vi "Mirror_Scan_Pixels_Main_V2.vi"() -> ()   [LabVIEW 2014]
uses:
  Pixel Scan Parameters.ctl
  MirrorModes.ctl
  Standard Action.ctl
  <vilib>/Analysis/baseanly.llb/Mean (DBL).vi
  <vilib>/Utility/file.llb/Write To Spreadsheet File (DBL).vi
  <vilib>/Utility/file.llb/Read From Spreadsheet File (DBL).vi
  <vilib>/Analysis/NI_AALBase.lvlib
panel:
  in  "Apply Zero":bool
  in  "Load V Map":bool
  in  "Load Modes":bool
  in  "Save Modes":bool
  in  "Save V Map":bool
  in  "Apply Flat":bool
  in  "Center Bias":bool
  in  "Exit":bool
  in  "Mirror Tab":T1(tab)
  in  "Mirror Modes":T2
  in  "Pixel Scan Parameters":T3={"Scan Start Pixel"=1, "Scan End Pixel"=1, "Pixel Start Value (-1 to 1)"=-0.5, "Pixel End Value (-1 to 1)"=0.5, "Number of Steps"=0.1}
  in  "Start Pixel Scan":bool
  out "Pixel Map (-1 to 1)":dbl[][](graph)
  # "Mode"
  # "Amount (nm)"
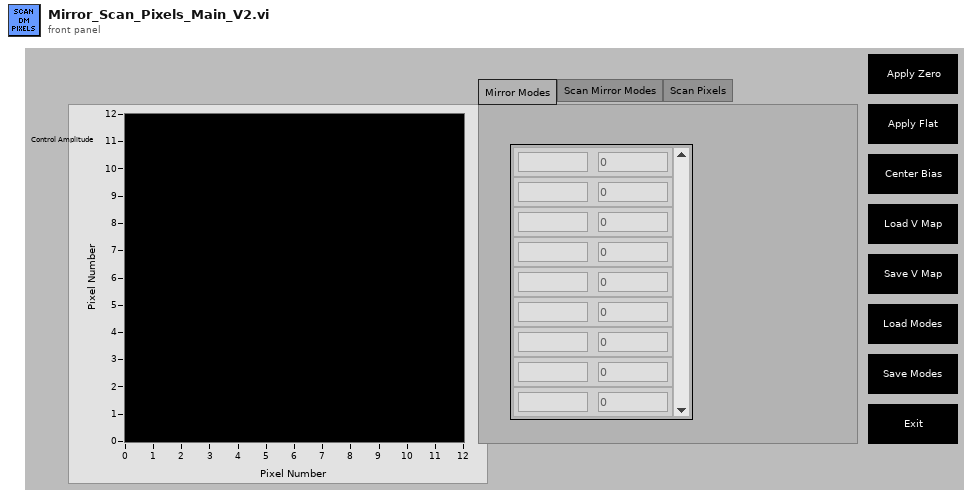
[diagram p1: front panel]
types:
  T1 = enum32{"Mirror Modes", "Scan Mirror Modes", "Scan Pixels"}
  T2 = typedef "MirrorModes.ctl" = cluster{"Mode":string, "Amplitude":dbl}[]
  T3 = typedef "Pixel Scan Parameters.ctl" = cluster{"Scan Start Pixel":i32, "Scan End Pixel":i32, "Pixel Start Value (-1 to 1)":dbl, "Pixel End Value (-1 to 1)":dbl, "Number of Steps":dbl}
  T4 = enum16{"Start Scan", "Reset Counter", "Write DM", "Get Image", "Update Count", "Exit"}
  T5 = typedef "Standard Action.ctl" = enum16{"Read", "Write"}
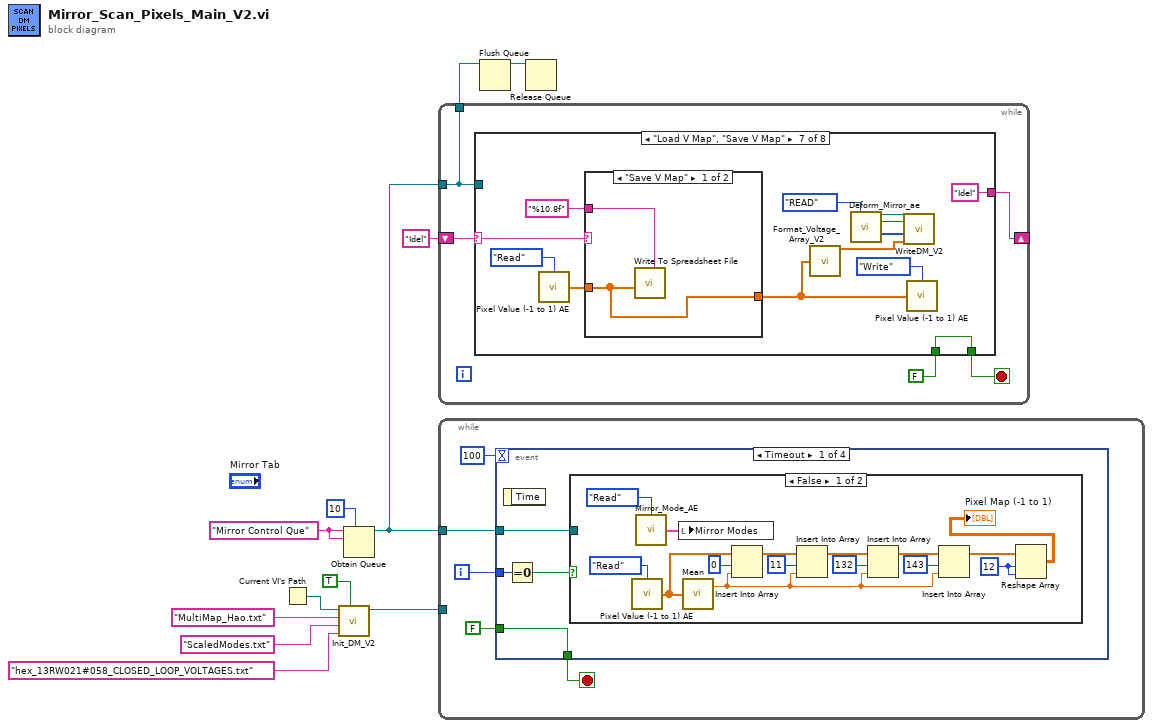
[diagram p0: block diagram]
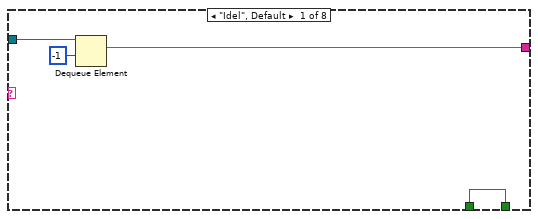
[diagram p2: hidden frame]
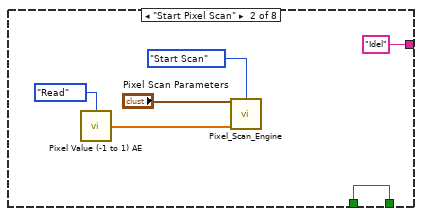
[diagram p3: hidden frame]
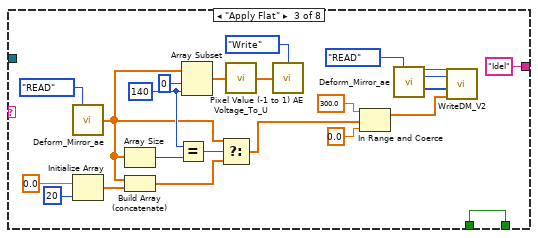
[diagram p4: hidden frame]
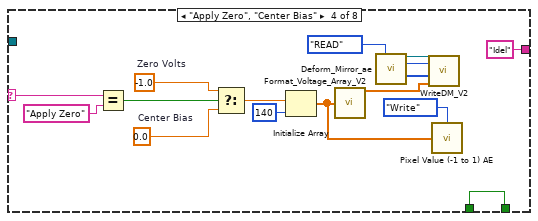
[diagram p5: hidden frame]
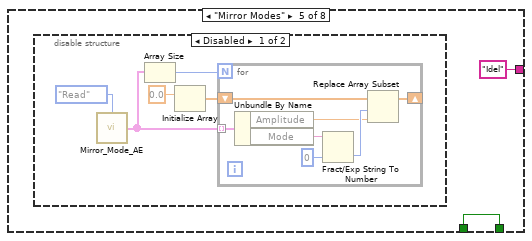
[diagram p6: hidden frame]
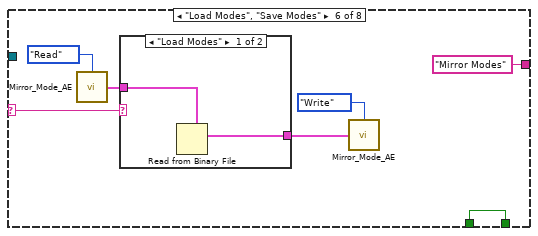
[diagram p8: hidden frame]
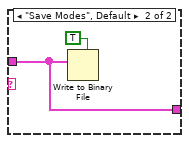
[diagram p9: hidden frame]
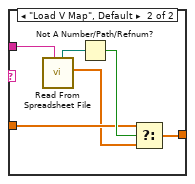
[diagram p10: hidden frame]
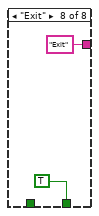
[diagram p11: hidden frame]
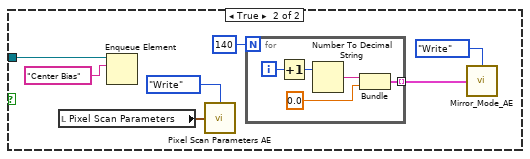
[diagram p12: hidden frame]
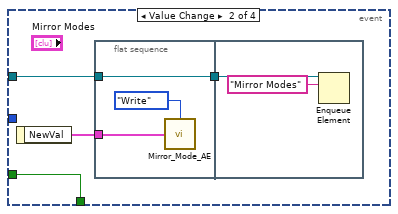
[diagram p13: hidden frame]
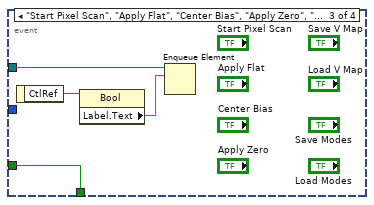
[diagram p14: hidden frame]
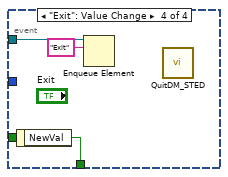
[diagram p15: hidden frame]
diagram:
  w12 = "Mirror Control Que" ("name (unnamed)")
  n1 = Current VI's Path() -> (path=w4:path)
  n2 = call "Init_DM_V2.vi"("BM Flat"=TRUE, "BM Flat File"="hex_13RW021#058_CLOSED_LOOP_VOLTAGES.txt" ("name or relative path"), "Mirror Modes File"="ScaledModes.txt" ("name or relative path"), "DM Mapping File"="MultiMap_Hao.txt" ("name or relative path"), "Base File Path"=w4) -> ("reference out"=w10:refnum<k7>)  [unwired: 6 in]
  n3 = Obtain Queue(max queue size (-1, unlimited)=10, name (unnamed)=w12, element data type=w12) -> (queue out=w6:refnum<queue>)  [unwired: 2 in, 2 out]
  n4 = while {
    tunnel: w6 -> [w13]
    shift-right: [w17] -> _
    shift-left: "Idel" ("name (unnamed)") -> [w16]
    tunnel: [w13] -> w9
    stop <- w15 stop-if-true
    n5 = case shown="\"Load V Map\", \"Save V Map\"" w16 {
      selector: w16 -> [_ _ _ w55 _ w83 w103 _]
      tunnel: w13 -> [w21 _ _ _ _ _ _ _]
      tunnel: [w19 "Idel" ("name (unnamed)") "Idel" ("name (unnamed)") "Idel" ("name (unnamed)") "Idel" ("name (unnamed)") "Mirror Modes" ("name (unnamed)") "Idel" ("name (unnamed)") "Exit" ("name (unnamed)")] -> w17
      tunnel: [w18 w27 w49 w66 w68 w87 w104 TRUE] -> w15
      tunnel: FALSE -> [w18 w27 w49 w66 w68 w87 w104 _]
      frame "Idel", Default {
        n6 = Dequeue Element(queue=w21, timeout in ms (-1)=-1) -> (element=w19:string)  [unwired: 1 in, 3 out]
      }
      frame "Start Pixel Scan" {
        n7 = call "Pixel Value (-1 to 1) AE.vi"("Action"=enum16{"Read", "Write"}."Read") -> ("Pixel Value (-1 to 1) Out"=w25:dbl[])  [unwired: 14 in]
        n8 = call "Pixel_Scan_Engine.vi"("Pixel Scan Parameters In"="Pixel Scan Parameters", "Action"=T4."Start Scan", "Initial Pixel Values (-1 to 1)"=w25) -> ()  [unwired: 13 in]
      }
      frame "Apply Flat" {
        w36 = 140 ("length")
        n9 = call "Deform_Mirror_ae.vi"("Enum"=enum16{"WRITE", "READ"}."READ") -> ("Flat Files Out"=w29:dbl[])  [unwired: 10 in, 4 out]
        n10 = Initialize Array(0.0 ("element"), 20 ("dimension size")) -> (w31:dbl[])
        n11 = Array Size(array=w29) -> (size(s)=w35:i32)
        n12 = Build Array (concatenate)(w29, w31) -> (w30:dbl[])
        n13 = Equal?(x=w36, y=w35) -> (x = y?=w34:bool)
        n14 = Array Subset(array=w29, index=0, length=w36) -> (w37:dbl[])
        n15 = Select(t=w29, s=w34, f=w30) -> (s? t:f=w28:dbl[])
        n16 = call "Voltage_To_U.vi"("Voltages In (Volts)"=w37) -> ("Pixel Value (-1 to 1)"=w39:dbl[])  [unwired: 14 in]
        n17 = call "Pixel Value (-1 to 1) AE.vi"("Action"=enum16{"Read", "Write"}."Write", "Pixel Value (-1 to 1)"=w39) -> ()  [unwired: 13 in, 1 out]
        n18 = In Range and Coerce(upper limit=300.0, x=w28, lower limit=0.0) -> (coerced(x)=w41:dbl[])  [unwired: 1 out]
        n19 = call "Deform_Mirror_ae.vi"("Enum"=enum16{"WRITE", "READ"}."READ") -> ("Refnum Out"=w47:refnum<k7>, "IDs Out"=w46:i32, "Multi Map Data Out"=w45:i32[])  [unwired: 10 in, 2 out]
        n20 = call "WriteDM_V2.vi"("reference in"=w47, "nDevId"=w46, "MultiDM  Mapping"=w45, "Voltage Array in"=w41) -> ()  [unwired: 2 in, 2 out]
      }
      frame "Apply Zero", "Center Bias" {
        w51 = -1.0  # Zero Volts
        w53 = 0.0  # Center Bias
        n21 = Equal?(x=w55, y="Apply Zero") -> (x = y?=w54:bool)
        n22 = Select(t=w51, s=w54, f=w53) -> (s? t:f=w52:dbl)
        n23 = Initialize Array(w52, 140 ("dimension size")) -> (w64:dbl[])
        n24 = call "Format_Voltage_Array_V2.vi"("Pixel Level (-1 to 1)"=w64) -> ("Voltage Array (Volts)"=w62:dbl[])  [unwired: 13 in, 1 out]
        n25 = call "Deform_Mirror_ae.vi"("Enum"=enum16{"WRITE", "READ"}."READ") -> ("Refnum Out"=w57:refnum<k7>, "IDs Out"=w58:i32, "Multi Map Data Out"=w59:i32[])  [unwired: 10 in, 2 out]
        n26 = call "WriteDM_V2.vi"("reference in"=w57, "nDevId"=w58, "MultiDM  Mapping"=w59, "Voltage Array in"=w62) -> ()  [unwired: 2 in, 2 out]
        n27 = call "Pixel Value (-1 to 1) AE.vi"("Action"=enum16{"Read", "Write"}."Write", "Pixel Value (-1 to 1)"=w64) -> ()  [unwired: 13 in, 1 out]
      }
      frame "Mirror Modes" {
        n28 = disable-structure shown="Disabled" {
          frame Disabled {
            n29 = call "Mirror_Mode_AE.vi"("Action"=Standard_Action."Read") -> ("Mirror Modes Out"=w72:T2)  [unwired: 14 in]
            n30 = Array Size(array=w72) -> (size(s)=w71:i32)
            n31 = Initialize Array(0.0 ("element")) -> (w69:dbl[])  [unwired: 1 in]
            n32 = for {
              N: w71 -> [_]
              tunnel: w72 -> [w80] mode=indexing
              shift-right: [w74] -> _
              shift-left: w69 -> [w75]
              n33 = Unbundle By Name(w80) -> ("Amplitude"=w76:dbl, "Mode"=w78:string)
              n34 = Fract/Exp String To Number(string=w78, default (0 dbl)=0) -> (number=w77:i32)  [unwired: 2 in, 1 out]
              n35 = Replace Array Subset(array=w75, new element=w76, index=w77) -> (w74:dbl[])
            }
          }
          frame Enabled {
          }
        }
      }
      frame "Load Modes", "Save Modes" {
        n36 = call "Mirror_Mode_AE.vi"("Action"=Standard_Action."Read") -> ("Mirror Modes Out"=w82:T2)  [unwired: 14 in]
        n37 = case shown="\"Load Modes\"" w83 {
          tunnel: w82 -> [w89 w90]
          tunnel: [w88 w90] -> w81
          frame "Load Modes" {
            n38 = Read from Binary File(5:w89) -> (2:w88:T2)  [unwired: 5 in, 3 out]
          }
          frame "Save Modes", Default {
            n39 = Write to Binary File(data=w90, 5:TRUE ("prepend array or string size? (T)")) -> ()  [unwired: 4 in, 3 out]
          }
        }
        n40 = call "Mirror_Mode_AE.vi"("Action"=Standard_Action."Write", "Mirror Modes In"=w81) -> ()  [unwired: 13 in, 1 out]
      }
      frame "Load V Map", "Save V Map" {
        n41 = call "Pixel Value (-1 to 1) AE.vi"("Action"=Standard_Action."Read") -> ("Pixel Value (-1 to 1) Out"=w101:dbl[])  [unwired: 14 in]
        n42 = case shown="\"Save V Map\"" w103 {
          tunnel: w101 -> [w105 w109]
          tunnel: "%10.8f" -> [w106 w112]
          tunnel: [w105 w107] -> w92
          frame "Save V Map" {
            n43 = call-poly <vilib>:"Write To Spreadsheet File.vi"("format (%.3f)"=w106, "1D data"=w105) -> ()  [unwired: 6 in, 1 out]
          }
          frame "Load V Map", Default {
            n44 = call-poly <vilib>:"Read From Spreadsheet File.vi"("format (%.3f)"=w112) -> ("first row"=w108:dbl[], "new file path (Not A Path if cancelled)"=w111:path)  [unwired: 6 in, 3 out]
            n45 = Not A Number/Path/Refnum?(number/path/refnum=w111) -> (NaN/Path/Refnum?=w110:bool)
            n46 = Select(t=w109, s=w110, f=w108) -> (s? t:f=w107:dbl[])
          }
        }
        n47 = call "Format_Voltage_Array_V2.vi"("Pixel Level (-1 to 1)"=w92) -> ("Voltage Array (Volts)"=w97:dbl[])  [unwired: 13 in, 1 out]
        n48 = call "Deform_Mirror_ae.vi"("Enum"=enum16{"WRITE", "READ"}."READ") -> ("Refnum Out"=w93:refnum<k7>, "IDs Out"=w94:i32, "Multi Map Data Out"=w95:i32[])  [unwired: 10 in, 2 out]
        n49 = call "WriteDM_V2.vi"("reference in"=w93, "nDevId"=w94, "MultiDM  Mapping"=w95, "Voltage Array in"=w97) -> ()  [unwired: 2 in, 2 out]
        n50 = call "Pixel Value (-1 to 1) AE.vi"("Action"=Standard_Action."Write", "Pixel Value (-1 to 1)"=w92) -> ()  [unwired: 13 in, 1 out]
      }
      frame "Exit" {
      }
    }
  }
  n51 = while {
    tunnel: w6 -> [w115]
    tunnel: w10 -> [_]
    i -> [w116]
    stop <- w119 stop-if-true
    n52 = event shown="[0] Timeout" {
      selector: _ -> [_ _ _ _]
      dyn-events: _ -> [_ _ _ _]
      timeout: 100 -> [_ _ _ _]
      tunnel: [w123 w154 w163 w166] -> w119
      tunnel: FALSE -> [w123 w154 w163 _]
      tunnel: w116 -> [w122 _ _ _]
      tunnel: w115 -> [w120 w152 w162 w165]
      event Timeout {
        n53 = event-data() -> ()  [unwired: 1 in, 1 out]
        n54 = Equal To 0?(x=w122) -> (x = 0?=w121:bool)
        n55 = case shown="False" w121 {
          tunnel: w120 -> [_ w145]
          frame False {
            w137 = 12 ("dimension size")
            n56 = call "Pixel Value (-1 to 1) AE.vi"("Action"=Standard_Action."Read") -> ("Pixel Value (-1 to 1) Out"=w138:dbl[])  [unwired: 14 in]
            n57 = call "Mirror_Mode_AE.vi"("Action"=Standard_Action."Read") -> ("Mirror Modes Out"=w125:T2)  [unwired: 14 in]
            n58 = local write "Mirror Modes"(w125) -> ()
            n59 = call-poly <vilib>:"Mean.vi"("X"=w138) -> ("mean"=w135:dbl)  [unwired: 1 out]
            n60 = Insert Into Array(array=w138, index=0, new element=w135) -> (w130:dbl[])
            n61 = Insert Into Array(array=w130, index=11, new element=w135) -> (w132:dbl[])
            n62 = Insert Into Array(array=w132, index=132, new element=w135) -> (w134:dbl[])
            n63 = Insert Into Array(array=w134, index=143, new element=w135) -> (w127:dbl[])
            n64 = Reshape Array(w127, w137, w137) -> (→"Pixel Map (-1 to 1)":dbl[][])
          }
          frame True {
            n65 = local read "Pixel Scan Parameters"() -> (w142:T3)
            n66 = Enqueue Element(queue=w145, element="Center Bias") -> ()  [unwired: 2 in, 3 out]
            n67 = call "Pixel Scan Parameters AE.vi"("Action"=enum16{"Write", "Read"}."Write", "Pixel Scan Parameters"=w142) -> ()  [unwired: 13 in, 1 out]
            n68 = for {
              N: 140 -> [_]
              tunnel: [w146] -> w139 mode=indexing
              i -> [w150]
              n69 = Increment(x=w150) -> (x+1=w149:i32)
              n70 = Number To Decimal String(number=w149) -> (decimal integer string=w148:string)  [unwired: 1 in]
              n71 = Bundle(w148, 0.0) -> (w146:cluster{string, dbl})  [unwired: 1 in]
            }
            n72 = call "Mirror_Mode_AE.vi"("Action"=Standard_Action."Write", "Mirror Modes In"=w139) -> ()  [unwired: 13 in, 1 out]
          }
        }
      }
      event Value Change {
        n73 = event-data() -> ("NewVal"=w153:T2)  [unwired: 1 in]
        n74 = flat-sequence {
          tunnel: w153 -> [w156]
          tunnel: w152 -> [w155]
          tunnel: [w155] -> w151
          tunnel: w151 -> [w159]
          frame #0 {
            n75 = call "Mirror_Mode_AE.vi"("Action"=Standard_Action."Write", "Mirror Modes In"=w156) -> ()  [unwired: 13 in, 1 out]
          }
          frame #1 {
            n76 = Enqueue Element(queue=w159, element="Mirror Modes") -> ()  [unwired: 2 in, 3 out]
          }
        }
      }
      event "Start Pixel Scan", "Apply Flat", "Center Bias", "Apply Zero", "Save V Map", "Save Modes", "Load Modes", "Load V Map": Value Change {
        n77 = event-data() -> ("CtlRef"=w161:refnum<vi>)  [unwired: 1 in]
        n78 = property class="Bool"(reference=w161) -> ("Label.Text"=w160:string)  [unwired: 1 in, 2 out]
        n79 = Enqueue Element(queue=w162, element=w160) -> ()  [unwired: 2 in, 3 out]
      }
      event "Exit": Value Change {
        n80 = event-data() -> ("NewVal"=w166:bool)  [unwired: 1 in]
        n81 = Enqueue Element(queue=w165, element="Exit") -> ()  [unwired: 2 in, 3 out]
        n82 = call "QuitDM_STED.vi"() -> ()  [unwired: 12 in]
      }
    }
  }
  n83 = Flush Queue(queue=w9) -> (queue out=w8:refnum<queue>)  [unwired: 1 in, 2 out]
  n84 = Release Queue(queue=w8) -> ()  [unwired: 2 in, 3 out]
